vi "LectFicLUT_IDL.vi"(0 "CheminFichierLUT":path) -> (1 "ImageLUT":picture, 2 "TabValLUT":u32[](array[numeric]))   [LabVIEW 2020]
doc: "Nom du VI : LectFicLUT_IDL.vi\n\nDescription : \nCe vi lit les données d'un fichier LUT (IDL) et dessine une LUT grâce à la fonction AffichageLUT. \n\nPrincipe : La fonction commence par lire un fichier sur le disque, les espaces et les retours chariot du fichier sont virés puis elle transforme la chaîne en tableau de couleurs avant de l'afficher. \n\nVariables d'entrée : CheminFichierLUT, tableau d'entiers non signés de 32 bits. Ce tableau représente la MUT à dessiner. \n\nVariables de sortie : \nTabValLUT, Tableau d'entiers non signés de 32 bits, ce tableau représente les couleurs de la LUT codées sur 24 bits. \nImageLUT, Image représentant la LUT. Cette image permet vérifier si la LUT chargée convient."
panel:
  out "Graphe d'intensité":dbl[][](graph)
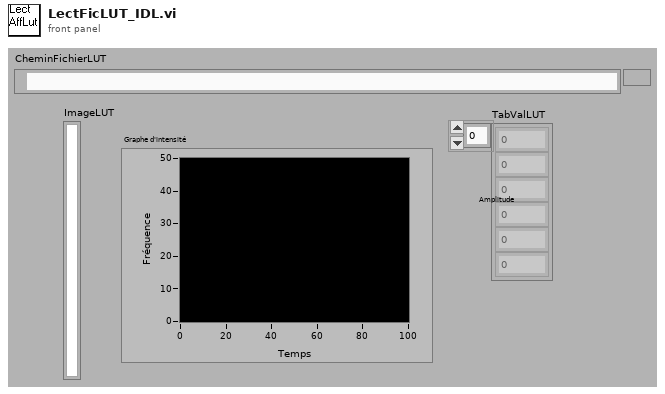
[diagram p1: front panel]
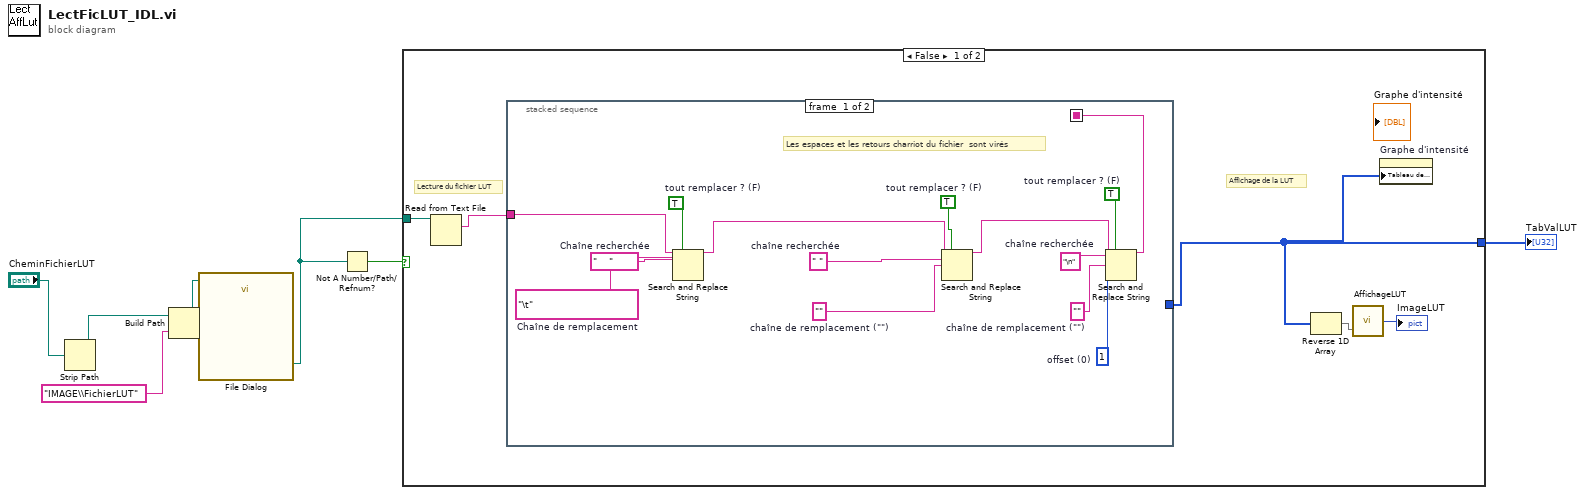
[diagram p0: block diagram]
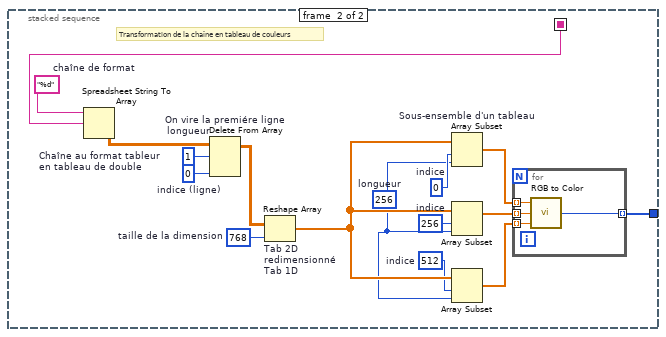
[diagram p2: hidden frame]
diagram:
  n1 = Strip Path(path="CheminFichierLUT") -> (stripped path=w5:path)  [unwired: 1 out]
  n2 = Build Path(base path=w5, name or relative path="IMAGE\\FichierLUT" ("name")) -> (appended path=w6:path)
  n3 = call "File Dialog"("start path"=w6) -> ("selected path"=w3:path)  [unwired: 11 in, 3 out]
  n4 = Not A Number/Path/Refnum?(number/path/refnum=w3) -> (NaN/Path/Refnum?=w2:bool)
  n5 = case shown="False" w2 {
    tunnel: w3 -> [w9 _]
    tunnel: [w8 _] -> w1
    frame False {
      # "Lecture du fichier LUT"
      # "Affichage de la LUT"
      n6 = Read from Text File(file (use dialog)=w9) -> (text=w10:string)  [unwired: 3 in, 3 out]
      n7 = stacked-sequence {
        seq-local: [w13 _] -> [_ w35]
        tunnel: w10 -> [w15 _]
        tunnel: [_ w28] -> w8
        frame #0 {
          w17 = TRUE  # tout remplacer ? (F)
          w18 = 1  # offset (0)
          w19 = ""  # chaîne de remplacement ("")
          w20 = "\n"  # chaîne recherchée
          w23 = "    "  # Chaîne recherchée
          w21 = "\t"  # Chaîne de remplacement
          w22 = TRUE  # tout remplacer ? (F)
          w24 = TRUE  # tout remplacer ? (F)
          w25 = ""  # chaîne de remplacement ("")
          w26 = " "  # chaîne recherchée
          # "Les espaces et les retours charriot du fichier  sont virés"
          n8 = Search and Replace String(replace all?=w22, input string=w15, search string=w23, replace string=w21) -> (result string=w16:string)  [unwired: 4 in, 3 out]
          n9 = Search and Replace String(replace all?=w24, input string=w16, search string=w26, replace string=w25) -> (result string=w14:string)  [unwired: 4 in, 3 out]
          n10 = Search and Replace String(replace all?=w17, input string=w14, search string=w20, replace string=w19, offset=w18) -> (result string=w13:string)  [unwired: 3 in, 3 out]
        }
        frame #1 {
          w29 = "%d"  # chaîne de format
          w32 = 1  # longueur
          w33 = 0  # indice (ligne)
          w36 = 512  # indice
          w37 = 256  # indice
          w38 = 256  # longueur
          w39 = 0  # indice
          w42 = 768  # taille de la dimension
          # "Transformation de la chaîne en tableau de couleurs"
          n11 = Spreadsheet String To Array "Chaîne au format tableur\nen tableau de double"(format string=w29, spreadsheet string=w35) -> (array=w34:dbl[][])  [unwired: 2 in]
          n12 = Delete From Array "On vire la premiére ligne"(array=w34, length=w32, index (col)=w33) -> (array with subset deleted=w41:dbl[][])  [unwired: 1 in, 1 out]
          n13 = Reshape Array "Tab 2D\nredimensionné \nTab 1D"(w41, w42) -> (w40:dbl[])
          n14 = Array Subset "Sous-ensemble d'un tableau"(array=w40, index=w39, length=w38) -> (w27:dbl[])
          n15 = Array Subset(array=w40, index=w37, length=w38) -> (w31:dbl[])
          n16 = Array Subset(array=w40, index=w36, length=w38) -> (w30:dbl[])
          n17 = for {
            tunnel: w27 -> [w46] mode=indexing
            tunnel: w31 -> [w45] mode=indexing
            tunnel: w30 -> [w44] mode=indexing
            tunnel: [w43] -> w28 mode=indexing
            n18 = call <vilib>:"RGB to Color.vi"("B"=w44, "G"=w45, "R"=w46) -> ("Color"=w43:u32)
          }
        }
      }
      n19 = Reverse 1D Array(array=w8) -> (reversed array=w11:u32[])
      n20 = call "AffichageLUT.vi"("Table de couleurs"=w11) -> ("LUT"=→"ImageLUT":picture)  [unwired: 1 in]
      n21 = property on="Graphe d'intensité" class="IntGraph (strict)"("Tableau de couleurs"=w8) -> ()  [unwired: 2 in, 2 out]
    }
    frame True {
    }
  }
  "TabValLUT" <- w1
